vi "Write Response String.vi"(8 "error in":errorcluster, 10 "message in":T1, 11 "lia rt in":refnum<class "Lock-In Amplifier Example RT.lvclass">) -> (0 "error out":errorcluster, 3 "lia rt out":refnum<class "Lock-In Amplifier Example RT.lvclass">)   [LabVIEW 2017, in "Lock-In Amplifier Example RT.lvclass"]
uses:
  Lock-In Amplifier Example RT.lvclass
  shared/Public/message.ctl
  Properties/Server_GET.vi
  server/RT FlexRIO Server TCP.lvclass
  shared/Lock-In Amplifier Example Shared.lvlib
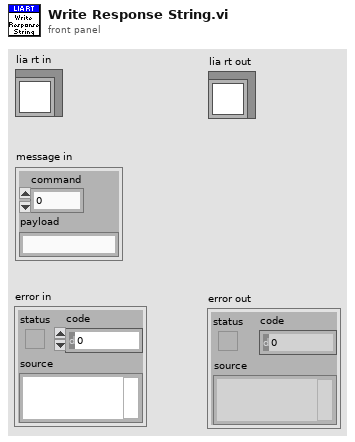
[diagram p1: front panel]
types:
  T1 = typedef "Lock-In Amplifier Example Shared.lvlib/message.ctl" = cluster{"command":u32, "payload":string}
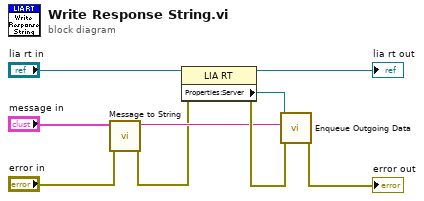
[diagram p0: block diagram]
diagram:
  n1 = call "Message to String.vi"("error in"="error in", "message in"="message in") -> ("error out"=w1:errorcluster, "string out"=w4:string)  [unwired: 8 in]
  n2 = property class="LIA RT"(reference="lia rt in", error in=w1) -> (reference out=→"lia rt out":refnum<class "Lock-In Amplifier Example RT.lvclass">, error out=w7:errorcluster, "Properties:Server"=w8:refnum<class "RT FlexRIO Server TCP.lvclass">)
  n3 = call "Enqueue Outgoing Data.vi"("error in"=w7, "string out"=w4, "server in"=w8) -> ("error out"=→"error out":errorcluster)  [unwired: 7 in, 1 out]
